vi "Stop Core.vi"(10 "final error code":i32, 11 "LSR Instrument in":refnum<class "LSR Instrument.lvclass">) -> (3 "LSR Instrument out":refnum<class "LSR Instrument.lvclass">)   [LabVIEW 2015, in "LSR Instrument.lvlib" / "LSR Instrument.lvclass"]
doc: "(<B>Filename</B>: Actor Framework.lvlib:Actor.lvclass:Stop Core.vi)\n\nDefines what the actor does before it stops. Use the <B>final error code</B> input to determine whether the actor shut down in response to an error.\n\nBy default, this method does nothing. A descendant class may override it to define behavior, such as shutting down any processes the actor initiated in its override of the Actor Core method."
uses:
  LSR Instrument.lvclass
  LSR Instrument.lvclass/LSR Instrument.ctl
  Actors/RDS Serial Instrument Actor/RDS Serial Instrument Actor.lvclass
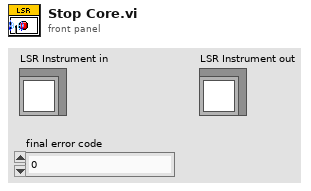
[diagram p1: front panel]
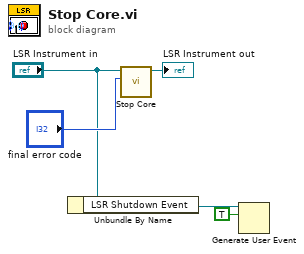
[diagram p0: block diagram]
diagram:
  n1 = Unbundle By Name("LSR Instrument in") -> ("LSR Shutdown Event"=w2:refnum<user-event>)
  n2 = call-parent "Stop Core.vi"("final error code"="final error code", "RDS Parent Actor in"="LSR Instrument in") -> ("RDS Parent Actor out"=→"LSR Instrument out":refnum<class "LSR Instrument.lvclass">)  [unwired: 9 in]
  n3 = Generate User Event(user event=w2, event data cluster=TRUE ("event data")) -> ()  [unwired: 2 in, 2 out]
